vi "solar_ui Listbox.vi"(7 "TargetLB":refnum<vi>, 8 "error in (no error)":errorcluster, 9 "Update LB Value? (F)":bool, 10 "Target":string, 11 "SOLAR Refnum":T1) -> (0 "error out":errorcluster, 1 "Listbox Value":i32, 3 "Active Target":T2)   [LabVIEW 2018]
doc: "This updates the SOLAR user interface target's listbox. The Target List displays the SOLAR Targets, Voyager Interfaces and QTimer References for the application."
uses:
  solar_ctl Target Global.ctl
  solar_ctl SOLAR Refnum.ctl
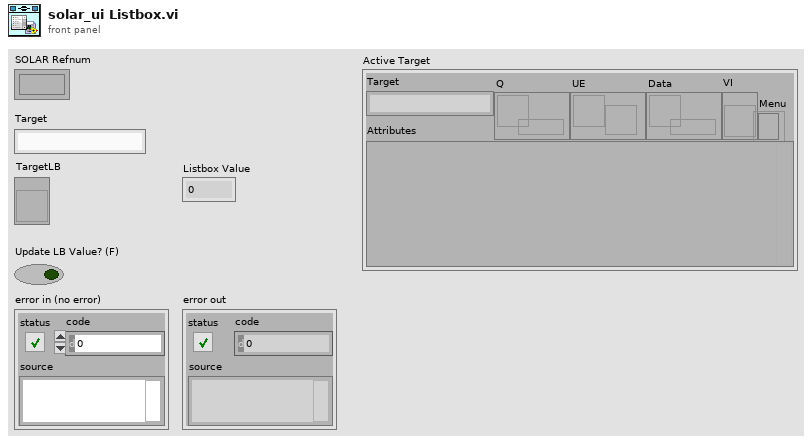
[diagram p1: front panel]
types:
  T1 = typedef "solar_ctl SOLAR Refnum.ctl" = refnum<k1>
  T2 = typedef "solar_ctl Target Global.ctl" = cluster{"Target":string, "Q":refnum<queue>, "UE":refnum<user-event>, "VI":refnum<vi>, "Menu":refnum<k9>, "Data":refnum<data-value>, "Attributes":variant}
  T3 = typedef "solar_ctl SOLAR Global.ctl" = cluster{"Targets":T2[], "AppDir":path, "solar.ini":path, "ConfigsDir":path, "CosmosDir":path, "LogsDir":path, "ExePath":path, "ExeVersion":string, "PartNum":string, "AppSetup":string, "Title":string, "Main.ini":path, "Temp.ini":path, "vSOLAR":string, "Splash.png":string, "SplashWait":i32, "SOLARUE":refnum<user-event>, "VoyagerRefnum":T4, "QTimerRefnum":T5}
  T4 = typedef "solar_voy_ctl Voyager Refnum.ctl" = refnum<k1>
  T5 = typedef "solar_qtimer_ctl Refnum.ctl" = refnum<k1>
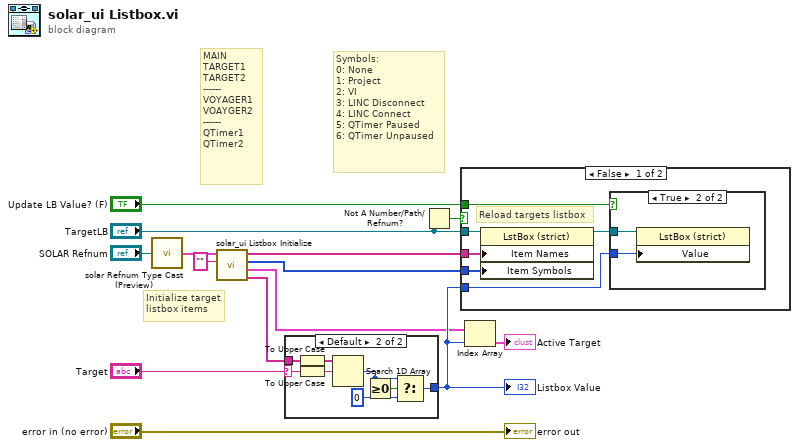
[diagram p0: block diagram]
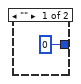
[diagram p4: hidden frame]
diagram:
  # "Initialize target\nlistbox items"
  # "Symbols:\n0: None\n1: Project\n2: VI\n3: LINC Disconnect\n4: LINC Connect\n5: QTimer Paused\n6: QTimer Unpaused"
  # "MAIN\nTARGET1\nTARGET2\n------\nVOYAGER1\nVOAYGER2\n------\nQTimer1\nQTimer2"
  n1 = call "solar Refnum Type Cast (Preview).vi"("Refnum"="SOLAR Refnum") -> ("SOLAR"=w7:T3)  [unwired: 8 in]
  n2 = call "solar_ui Listbox Initialize.vi"("Selected Listbox Item"="", "SOLAR"=w7) -> ("Visible Target Names"=w2:string[], "Visible Targets"=w3:T2[], "TargetLB Symbols"=w10:i32[], "TargetLB Names"=w11:string[])  [unwired: 4 in, 2 out]
  n3 = case shown="Default" "Target" {
    selector: "Target" -> [_ w17]
    tunnel: [0 ("t") w21] -> w5
    tunnel: w2 -> [_ w18]
    frame "" {
    }
    frame Default {
      n4 = To Upper Case(1:w18) -> (0:w20:string[])
      n5 = To Upper Case(1:w17) -> (0:w19:string)
      n6 = Search 1D Array(1D array=w20, element=w19) -> (index of element=w16:i32)  [unwired: 1 in]
      n7 = Greater Or Equal To 0?(x=w16) -> (x >= 0?=w23:bool)
      n8 = Select(t=w16, s=w23, f=0 ("t")) -> (s? t:f=w21:i32)
    }
  }
  "Listbox Value" <- w5
  n9 = Not A Number/Path/Refnum?(number/path/refnum="TargetLB") -> (NaN/Path/Refnum?=w13:bool)
  n10 = case shown="False" w13 {
    tunnel: "TargetLB" -> [w29 _]
    tunnel: w5 -> [w25 _]
    tunnel: w11 -> [w28 _]
    tunnel: w10 -> [w27 _]
    tunnel: "Update LB Value? (F)" -> [w24 _]
    frame False {
      # "Reload targets listbox"
      n11 = property class="LstBox (strict)"(reference=w29, "Item Names"=w28, "Item Symbols"=w27) -> (reference out=w26:refnum<vi>)  [unwired: 1 in, 1 out]
      n12 = case shown="True" w24 {
        tunnel: w26 -> [_ w31]
        tunnel: w25 -> [_ w30]
        frame False {
        }
        frame True {
          n13 = property class="LstBox (strict)"(reference=w31, "Value"=w30) -> ()  [unwired: 1 in, 2 out]
        }
      }
    }
    frame True {
    }
  }
  n14 = Index Array(array=w3, index=w5) -> (element=→"Active Target":T2)
  "error out" <- "error in (no error)"
